vi "Set Lower-HigherTravel Limit.vi"(4 "Travel Direction":T2, 8 "error in (no error)":errorcluster, 9 "Travel Units":T1, 10 "Limit":dbl format="%.3f", 11 "Force Test Stand in":refnum<class "Force Test Stand.lvclass">) -> (0 "error out":errorcluster, 3 "Force Test Stand out":refnum<class "Force Test Stand.lvclass">)   [LabVIEW 2018, in "Force Test Stand.lvlib" / "Force Test Stand.lvclass"]
uses:
  Force Test Stand.lvclass
  Custom Controls/Travel Direction.ctl
  Custom Controls/Travel Units.ctl
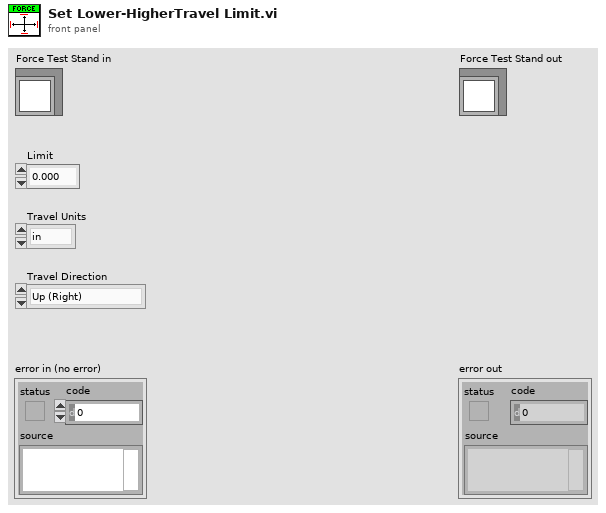
[diagram p1: front panel]
types:
  T1 = typedef "Force Test Stand.lvlib/Force Test Stand.lvclass/Travel Units.ctl" = enum16{"in", "mm"}
  T2 = typedef "Force Test Stand.lvlib/Force Test Stand.lvclass/Travel Direction.ctl" = enum16{"Up (Right)", "Down (Left)"}
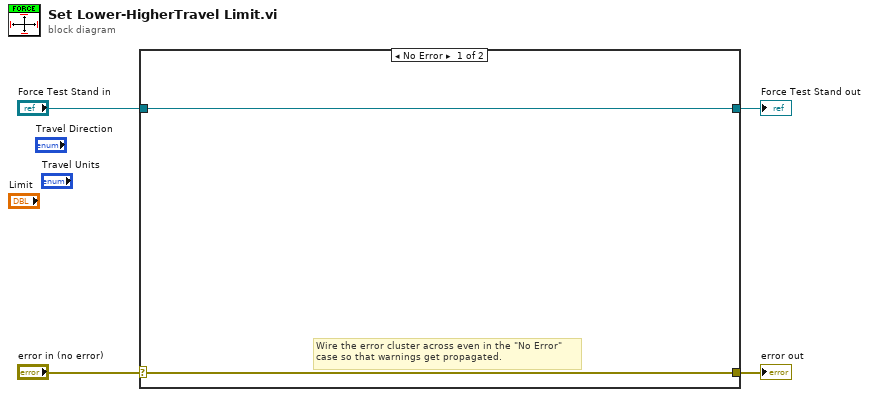
[diagram p0: block diagram]
diagram:
  n1 = case shown="No Error" "error in (no error)" {
    selector: "error in (no error)" -> [w5 w8]
    tunnel: [w5 w8] -> w3
    tunnel: [w6 w7] -> w1
    tunnel: "Force Test Stand in" -> [w6 w7]
    frame No Error {
      # "Wire the error cluster across even in the \"No Error\"\ncase so that warnings get propagated."
    }
    frame Error {
    }
  }
  "error out" <- w3
  "Force Test Stand out" <- w1
